vi "FTW-JSON-SerializeAndDestroy.vi"(0 "JSON Object":refnum<data-value>, 11 "error in":errorcluster) -> (6 "JSON String (UTF-8)":string, 15 "error out":errorcluster)   [LabVIEW 2014]
uses:
  core/FTW-JSON-Core-Structure.ctl
  lib/FTW-LibraryFilepath.vi
  error/FTW-ERR-ThrowGenericError.vi
  error/FTW-ERR-ThrowError.vi
  error/FTW-ERR-CallChain.vi
  string/FTW-STR-ReplaceWhitespace.vi
panel:
  # "Inputs"
  # "Outputs"
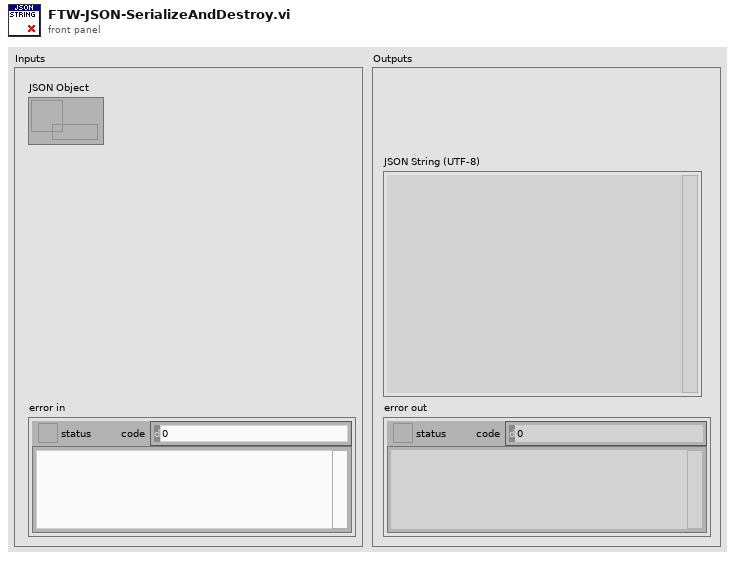
[diagram p1: front panel]
types:
  T1 = typedef "FTW-JSON-Core-Structure.ctl" = cluster{"JSON Object":i64, "Encoding Flags":i64, "Decoding Flags":i64}
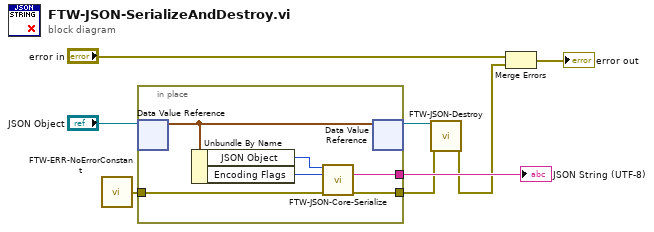
[diagram p0: block diagram]
diagram:
  n1 = call "FTW-ERR-NoErrorConstant.vi"() -> ("no error"=w1:errorcluster)
  n2 = in-place {
    in-place-border: [w14] -> w5
    in-place-border: [w13] -> w7
    in-place-border: w1 -> [w9]
    n3 = in-place-dvr #1("JSON Object") -> (w12:T1)  [unwired: 1 out]
    n4 = Unbundle By Name(w12) -> ("JSON Object"=w11:i64, "Encoding Flags"=w10:i64)
    n5 = call "FTW-JSON-Core-Serialize.vi"("JSON Object"=w11, "Encoding Flags"=w10, "error in"=w9) -> ("JSON String (UTF-8)"=w13:string, "error out"=w14:errorcluster)  [unwired: 10 in, 1 out]
    n6 = in-place-dvr #1(w12) -> (w6:refnum<data-value>)  [unwired: 1 out]
  }
  "JSON String (UTF-8)" <- w7
  n7 = call "FTW-JSON-Destroy.vi"("JSON Object"=w6, "error in"=w5) -> ("error out"=w3:errorcluster)  [unwired: 13 in]
  n8 = Merge Errors("error in", w3) -> (→"error out":errorcluster)
